vi "sigmoid.vi"(9 "t":dbl) -> (1 "S(t)":dbl)   [LabVIEW 2014]
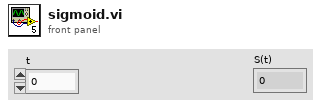
[diagram p1: front panel]
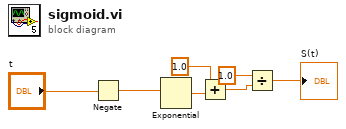
[diagram p0: block diagram]
diagram:
  n1 = Negate(x="t") -> (-x=w4:dbl)
  n2 = Exponential(1:w4) -> (0:w3:dbl)
  n3 = Add(x=1.0, y=w3) -> (x+y=w2:dbl)
  n4 = Divide(x=1.0, y=w2) -> (x/y=→"S(t)":dbl)
